vi "parse buttons.vi"(8 "error in (no error)":errorcluster, 11 "control\ncluster":T1) -> (0 "error out":errorcluster, 3 "control\ncluster out":T1)   [LabVIEW 2023]
uses:
  ctrl defs/ctrl controllers.ctl
  ctrl defs/ctrl DRIVING FRAME selector.ctl
  ctrl defs/ctrl FRONT FACE selector.ctl
  Global odometry.vi
panel:
  out "Button Pressed?":bool
  in  "button for\nAPRIL TAGS":i32=4
  out "Buttons":bool[](array[boolean])
  out "POVs":i16[](array[numeric])
  out "Axes":dbl[](array[numeric])
  in  "button for\nfront/rear\ndrive direction":i32=7
  in  "button for\nROBO/FLD\ncentric drive":i32=6
  in  "notes":string="Joystick 0 - pilot\n\ntoggle between robo-centric and field-centric driving\n\ntoggle between front (intake) and rear (shooter) sides\n\ntoggle APRIL TAGS\n\nNOTE: labels on joystick are labeled 1-12 but programmed 0-11"
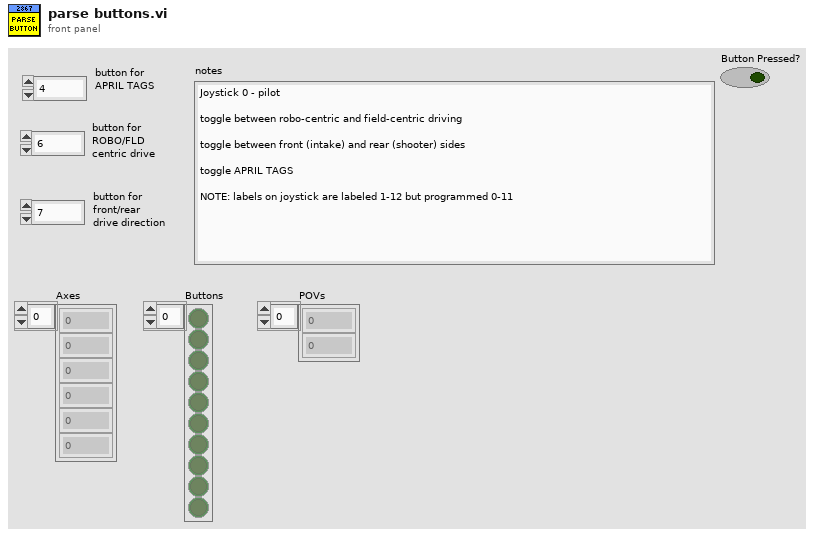
[diagram p1: front panel]
types:
  T1 = typedef "ctrl controllers.ctl" = cluster{"Axes":dbl[], "Buttons":bool[], "POVs":i16[]}
  T2 = typedef "ctrl FRONT FACE selector.ctl" = enum16{"intake side", "shooter side"}
  T3 = typedef "ctrl DRIVING FRAME selector.ctl" = enum16{"ROBO-centric", "FLD-centric"}
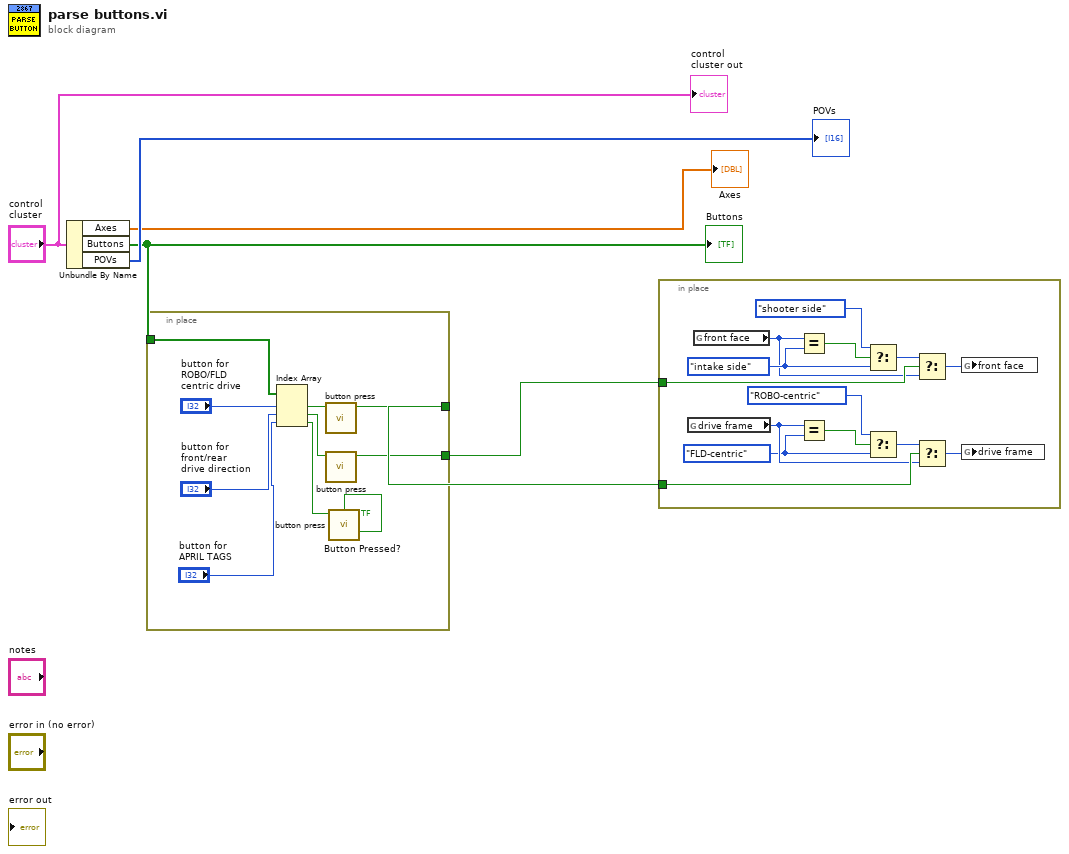
[diagram p0: block diagram]
diagram:
  n1 = Unbundle By Name("control\ncluster") -> ("Axes"=→"Axes":dbl[], "Buttons"=w2:bool[], "POVs"=→"POVs":i16[])
  "Buttons" <- w2
  n2 = in-place {
    in-place-border: w2 -> [w16]
    in-place-border: [w11] -> w5
    in-place-border: [w10] -> w4
    n3 = Index Array(array=w16, index #1="button for\nROBO/FLD\ncentric drive", index #2="button for\nfront/rear\ndrive direction", index #3="button for\nAPRIL TAGS") -> (element #1=w13:bool, element #2=w12:bool, element #3=w8:bool)
    n4 = call "button press.vi"("button IN"=w13) -> ("Button Pressed?"=w11:bool)  [unwired: 10 in]
    n5 = call "button press.vi"("button IN"=w12) -> ("Button Pressed?"=w10:bool)  [unwired: 10 in]
    n6 = call "button press.vi"("button IN"=w8) -> ("Button Pressed?"=→"Button Pressed?":bool)  [unwired: 10 in]
  }
  n7 = in-place {
    in-place-border: w5 -> [w29]
    in-place-border: w4 -> [w27]
    w20 = ctrl_FRONT_FACE_selector."intake side" ("front face")
    w22 = ctrl_DRIVING_FRAME_selector."FLD-centric" ("drive frame")
    n8 = global read "Global odometry.vi" "drive frame"() -> (w26:T3)
    n9 = global read "Global odometry.vi" "front face"() -> (w18:T2)
    n10 = Equal?(x=w18, y=w20) -> (x = y?=w21:bool)
    n11 = Equal?(x=w26, y=w22) -> (x = y?=w25:bool)
    n12 = Select(t=ctrl_FRONT_FACE_selector."shooter side" ("front face"), s=w21, f=w20) -> (s? t:f=w17:T2)
    n13 = Select(t=ctrl_DRIVING_FRAME_selector."ROBO-centric" ("drive frame"), s=w25, f=w22) -> (s? t:f=w23:T3)
    n14 = Select(t=w17, s=w27, f=w18) -> (s? t:f=w28:T2)
    n15 = Select(t=w23, s=w29, f=w26) -> (s? t:f=w30:T3)
    n16 = global write "Global odometry.vi" "front face"(w28) -> ()
    n17 = global write "Global odometry.vi" "drive frame"(w30) -> ()
  }
  "control\ncluster out" <- "control\ncluster"
